vi "Terminate.vi"(8 "error in (no error)":errorcluster, 10 "Message in":refnum<class "TerminateMessage.lvclass">, 11 "StageSPIM in":refnum<class "StageSPIM.lvclass">) -> (0 "error out":errorcluster, 3 "StageSPIM out":refnum<class "StageSPIM.lvclass">)   [LabVIEW 2012, in "StageSPIM.lvclass"]
doc: "This member function is called when the statemachine in the run.vi receives an 'terminate' command. It closes the RabbitMQ connection. \n\nOverride this member function in your derived class to release all previously acquired resources (but don't forget to call the parent method). If your component has subcomponents, they count as resources, and you have to release them by calling their own terminate functions."
uses:
  StageSPIM.lvclass
  <vilib>/Distrio/Murmex/Murmex/Murmex.lvclass
  <vilib>/Distrio/Murmex/TerminateMessage/TerminateMessage.lvclass
panel:
  out "Array":bool[](array[boolean])
  # "This method is called when the TERMINATE\ntrigger is sent. \n\nOverride this method when your component needs to\nrespond to this trigger. \n\nCall parent for proper implementation"
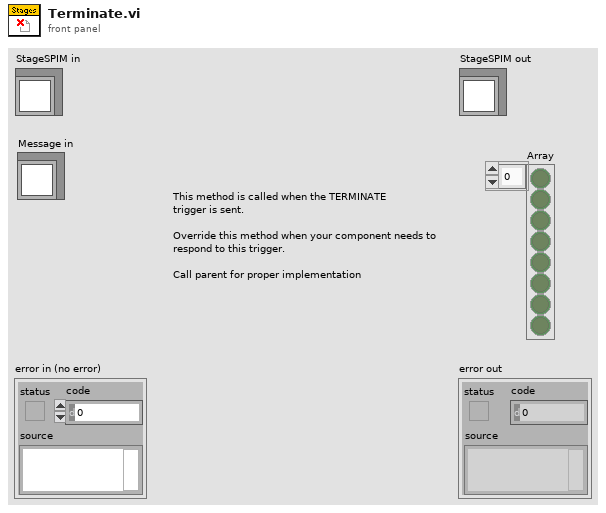
[diagram p1: front panel]
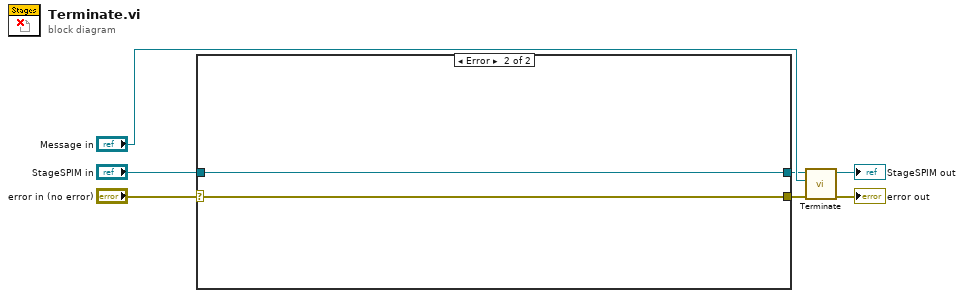
[diagram p0: block diagram]
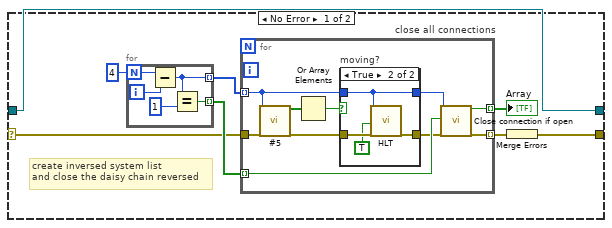
[diagram p2: hidden frame]
diagram:
  n1 = case shown="Error" "error in (no error)" {
    selector: "error in (no error)" -> [w10 w37]
    tunnel: [w9 w37] -> w5
    tunnel: "StageSPIM in" -> [w8 w38]
    tunnel: [w8 w38] -> w1
    frame No Error {
      # "create inversed system list\nand close the daisy chain reversed"
      n2 = for {
        N: 4 -> [w20]
        tunnel: [w18] -> w13 mode=indexing
        tunnel: [w16] -> w12 mode=indexing
        i -> [w19]
        n3 = Subtract(x=w20, y=w19) -> (x-y=w18:i32)
        n4 = Equal?(x=w18, y=1) -> (x = y?=w16:bool)
      }
      n5 = for "close all connections" {
        tunnel: w13 -> [w26] mode=indexing
        tunnel: w12 -> [w30] mode=indexing
        tunnel: [w29] -> w15 mode=indexing
        tunnel: w10 -> [w25]
        tunnel: [w28] -> w14 mode=indexing
        n6 = call "#5.vi"("System no."=w26, "error in"=w25) -> ("Axis moving?"=w23:bool[], "error out"=w24:errorcluster)  [unwired: 16 in]
        n7 = Or Array Elements(Boolean array=w23) -> (logical OR=w22:bool)
        n8 = case "moving?" shown="True" w22 {
          tunnel: [w31 w36] -> w27
          tunnel: w26 -> [w32 w33]
          tunnel: w24 -> [w31 w35]
          tunnel: [w32 w33] -> w21
          frame False {
          }
          frame True {
            n9 = call "HLT.vi"("System no."=w33, "All axes?"=TRUE ("all axes"), "error in"=w35) -> ("error out"=w36:errorcluster)  [unwired: 16 in]
          }
        }
        n10 = call "Close connection if open.vi"("System no."=w21, "Close DaisyChain"=w30, "error in"=w27) -> ("Was connected?"=w29:bool, "error out"=w28:errorcluster)  [unwired: 15 in]
      }
      "Array" <- w15
      n11 = Merge Errors(w14) -> (w9:errorcluster)
    }
    frame Error {
    }
  }
  n12 = call-parent "Terminate.vi"("error in (no error)"=w5, "Message in"="Message in", "Murmex in"=w1) -> ("error out"=→"error out":errorcluster, "Murmex out"=→"StageSPIM out":refnum<class "StageSPIM.lvclass">)  [unwired: 7 in]
